vi "lib Timestamp to Unix Time.vi"(8 "error in (no error)":errorcluster, 11 "Time Stamp":timestamp) -> (0 "error out":errorcluster, 3 "Unix Time":dbl)   [LabVIEW 2011]
panel:
  out "time stamp":timestamp format="%<%H:%M:%S\n%x>T"
  in  "Unix Basetime":timestamp=timestamp(2082844800 s since 1904-01-01)
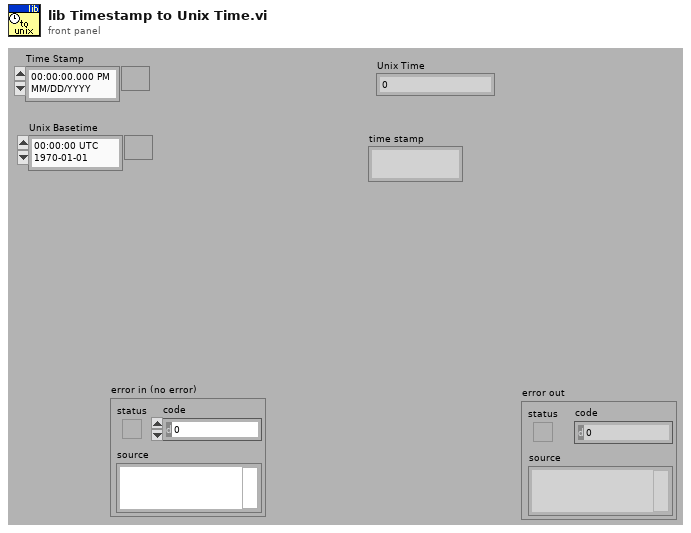
[diagram p1: front panel]
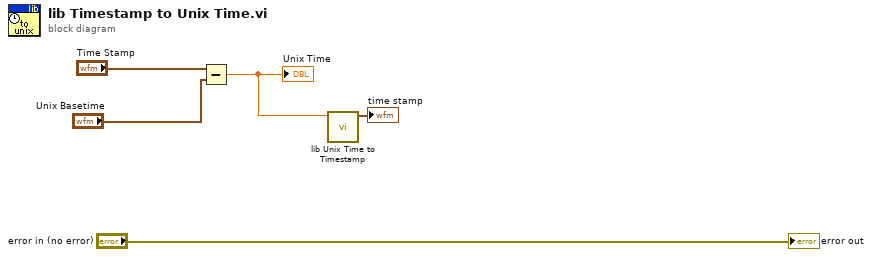
[diagram p0: block diagram]
diagram:
  n1 = Subtract(x="Time Stamp", y="Unix Basetime") -> (x-y=w2:dbl)
  "Unix Time" <- w2
  n2 = call "lib Unix Time to Timestamp.vi"("unix timestamp"=w2) -> ("time stamp"=→"time stamp":timestamp)  [unwired: 9 in, 1 out]
  "error out" <- "error in (no error)"
